vi "SetToString.vi"(0 "reference in":refnum<class "G#RemoteProxy.lvclass">, 2 "to string":string, 5 "error in (no error)":errorcluster) -> (14 "reference out":refnum<class "G#RemoteProxy.lvclass">, 19 "error out":errorcluster)   [LabVIEW 2017, in "G#RemoteProxy.lvclass"]
doc: "Sets ToString."
uses:
  G#RemoteProxy.lvclass
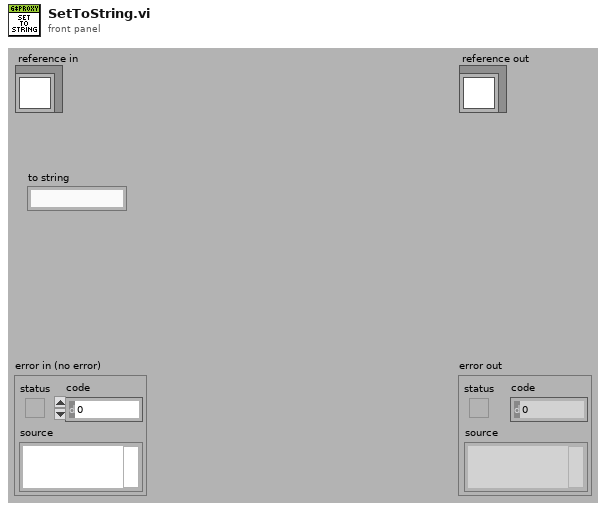
[diagram p1: front panel]
types:
  T1 = typedef "G#RemoteProxy.lvclass/ObjectAttributesRef.ctl" = refnum<data-value>
  T2 = typedef "G#RemoteProxy.lvclass/ObjectAttributesProxy.ctl" = cluster{"class hierarchy":T3[], "class name":string, "lvlib hierarchy":string[], "full class name":string, "id":u32, "owner":string, "RemoteRef":refnum<class "G#Object.lvclass">, "object name":string, "attributes":variant[], "connection ID":refnum<k5>, "address":u32, "occurrence":refnum<k4>, "ProxyClassRef":refnum<class "G#RemoteProxy.lvclass">, "InMemory?":bool, "ToString":string}
  T3 = typedef "G#Object.lvclass/G#Object_ClassHierarchy.ctl" = cluster{"ClassName":string, "FullClassName":string, "ClassPath":path, "IsLeaf":bool}
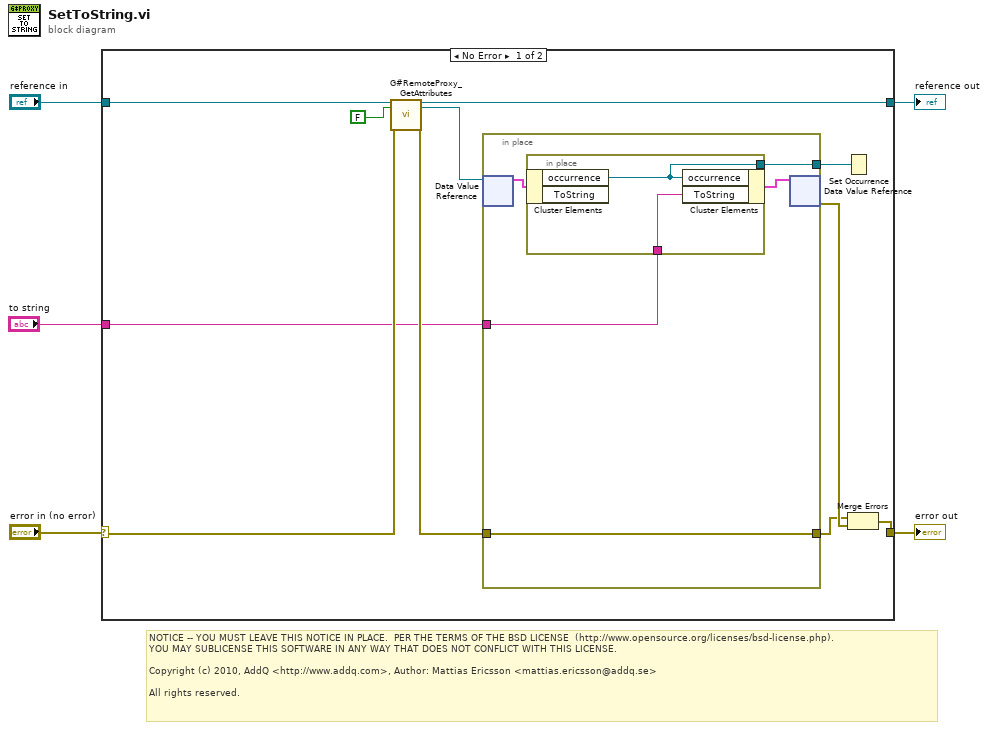
[diagram p0: block diagram]
diagram:
  # "NOTICE -- YOU MUST LEAVE THIS NOTICE IN PLACE.  PER THE TERMS OF THE BSD LICENSE  (http://www.opensource.org/licenses/bsd-license.php).\nYOU MAY SUBLICENSE THIS SOFTWARE IN ANY WAY THAT DOES NOT CONFLICT WITH THIS LICENSE.\n\nCopyright (c) 2010, AddQ <http://www.addq.com>, Author: Mattias Ericsson <mattias.ericsson@addq.se>\n\nAll rights reserved."
  n1 = case shown="No Error" "error in (no error)" {
    selector: "error in (no error)" -> [w11 w25]
    tunnel: [w16 w25] -> w4
    tunnel: [w9 w24] -> w2
    tunnel: "reference in" -> [w13 w24]
    tunnel: "to string" -> [w7 _]
    frame No Error {
      n2 = call "G#RemoteProxy_GetAttributes.vi"("reference in"=w13, "return data? (T)"=FALSE, "error in (no error)"=w11) -> ("reference out"=w9:refnum<class "G#RemoteProxy.lvclass">, "attributes ref"=w8:T1, "error out"=w10:errorcluster)  [unwired: 13 in, 1 out]
      n3 = in-place {
        in-place-border: w10 -> [w19]
        in-place-border: [w19] -> w14
        in-place-border: w7 -> [w18]
        in-place-border: [w17] -> w6
        n4 = in-place-dvr #1(w8) -> (w20:T2)  [unwired: 1 out]
        n5 = in-place {
          in-place-border: w18 -> [w23]
          in-place-border: [w22] -> w17
          n6 = in-place-cluster #2(w20) -> ("occurrence"=w22:refnum<k4>)  [unwired: 1 out]
          n7 = in-place-cluster #2("occurrence"=w22, "ToString"=w23) -> (w21:T2)
        }
        n8 = in-place-dvr #1(w21) -> (w15:errorcluster)  [unwired: 1 out]
      }
      n9 = Set Occurrence(w6) -> ()
      n10 = Merge Errors(w14, w15) -> (w16:errorcluster)
    }
    frame Error {
    }
  }
  "error out" <- w4
  "reference out" <- w2
